vi "csvNameGenerate.vi"(0 "User Name":string, 1 "time stamp":timestamp, 5 "Short Description":string, 7 "Threshold Value":u16, 9 "Acquisition Period":dbl, 11 "error in":errorcluster) -> (3 "Dump file path":path, 4 "Byte Stream File out":refnum<file>, 6 "File Name":string, 15 "error out":errorcluster)   [LabVIEW 2019]
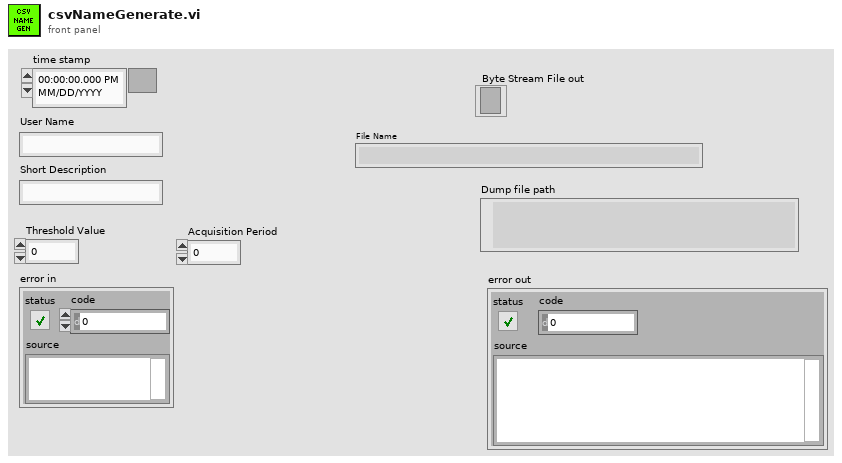
[diagram p1: front panel]
types:
  T1 = enum16{"open", "replace", "create", "open or create", "replace or create", "replace or create with confirmation"}
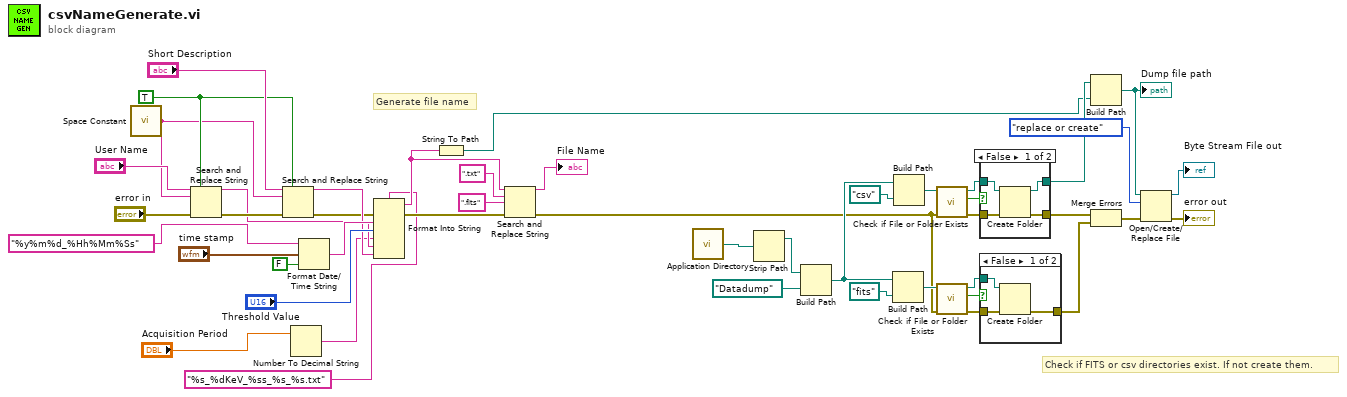
[diagram p0: block diagram]
diagram:
  w24 = TRUE ("replace all? (F)")
  # "Check if FITS or csv directories exist. If not create them."
  # "Generate file name"
  n1 = call <vilib>:"Space Constant.vi"() -> ("String"=w23:string)
  n2 = Search and Replace String(replace all?=w24, input string="User Name", search string=w23, error in="error in") -> (result string=w26:string, error out=w29:errorcluster)  [unwired: 4 in, 2 out]
  n3 = Search and Replace String(replace all?=w24, input string="Short Description", search string=w23, error in=w29) -> (result string=w30:string, error out=w28:errorcluster)  [unwired: 4 in, 2 out]
  n4 = Number To Decimal String(number="Acquisition Period") -> (decimal integer string=w25:string)  [unwired: 1 in]
  n5 = Format Date/Time String(time format string (%c)="%y%m%d_%Hh%Mm%Ss", seconds (now)="time stamp", UTC format=FALSE) -> (date/time string=w46:string)
  n6 = Format Into String(format string="%s_%dKeV_%ss_%s_%s.txt", error in=w28, w46, "Threshold Value", w25, w26, w30) -> (resulting string=w36:string, error out=w32:errorcluster)  [unwired: 1 in]
  n7 = String To Path(string=w36) -> (path=w15:path)
  n8 = Search and Replace String(input string=w36, search string=".txt", replace string=".fits", error in=w32) -> (result string=→"File Name":string, error out=w10:errorcluster)  [unwired: 4 in, 2 out]
  n9 = call <vilib>:"Application Directory.vi"() -> ("Application Directory"=w2:path)
  n10 = Strip Path(path=w2) -> (stripped path=w1:path)  [unwired: 1 out]
  n11 = Build Path(base path=w1, name or relative path=path "Datadump" ("base path")) -> (appended path=w12:path)
  n12 = Build Path(base path=w12, name or relative path=path "fits" ("base path")) -> (appended path=w11:path)
  n13 = Build Path(base path=w12, name or relative path=path "csv" ("base path")) -> (appended path=w17:path)
  n14 = call <vilib>:"Check if File or Folder Exists.vi"("error in (no error)"=w10, "path"=w17) -> ("error out"=w22:errorcluster, "file or folder exists?"=w20:bool, "dup path"=w21:path)  [unwired: 7 in]
  n15 = call <vilib>:"Check if File or Folder Exists.vi"("error in (no error)"=w10, "path"=w11) -> ("error out"=w8:errorcluster, "file or folder exists?"=w4:bool, "dup path"=w9:path)  [unwired: 7 in]
  n16 = case shown="False" w20 {
    tunnel: w22 -> [w50 w51]
    tunnel: w21 -> [w49 w52]
    tunnel: [w48 w52] -> w16
    tunnel: [w47 w51] -> w6
    frame False {
      n17 = Create Folder(path (use dialog)=w49, error in=w50) -> (created path=w48:path, error out=w47:errorcluster)  [unwired: 1 in, 1 out]
    }
    frame True {
    }
  }
  n18 = case shown="False" w4 {
    tunnel: w8 -> [w55 w56]
    tunnel: w9 -> [w54 _]
    tunnel: [w53 w56] -> w7
    frame False {
      n19 = Create Folder(path (use dialog)=w54, error in=w55) -> (error out=w53:errorcluster)  [unwired: 1 in, 2 out]
    }
    frame True {
    }
  }
  n20 = Build Path(base path=w16, name or relative path=w15) -> (appended path=w14:path)
  "Dump file path" <- w14
  n21 = Merge Errors(w6, w7) -> (w5:errorcluster)
  n22 = Open/Create/Replace File(file path (use dialog)=w14, error in=w5, operation (0:open)=T1."replace or create") -> (refnum out=→"Byte Stream File out":refnum<file>, error out=→"error out":errorcluster)  [unwired: 3 in, 1 out]
